vi "Clear Bit.vi"(10 "bit index":u8, 11 "value in":u8 format="%08b") -> (3 "value out":u8 format="%08b")   [LabVIEW 2017, in "DSF Core.lvlib" / "Buffer Converter.lvclass"]
uses:
  Buffer Converter.lvclass
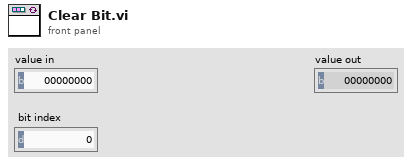
[diagram p1: front panel]
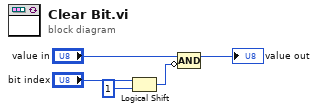
[diagram p0: block diagram]
diagram:
  n1 = Logical Shift(y="bit index", x=u8 1) -> (x << y=w1:u8)
  n2 = Compound Arithmetic op=AND("value in", invert w1) -> (→"value out":u8)
